vi "OAT Get Missing Pulses.vi"(3 "pulse positions":dbl[](array[numeric]) format="%.2f") -> (0 "pulses inserted":i32, 1 "modified pulse positions":dbl[](array[numeric]) format="%.2f")   [LabVIEW 2017, in "SoundVib_TachProcess.lvlib"]
uses:
  <vilib>/addons/Sound and Vibration/Order Analysis/Tach Process/SoundVib_TachProcess.lvlib
  <vilib>/Analysis/NI_AALBase.lvlib
panel:
  # "Get Missing Pules"
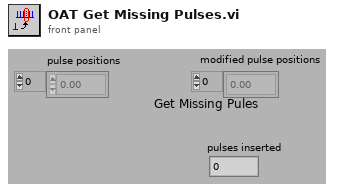
[diagram p1: front panel]
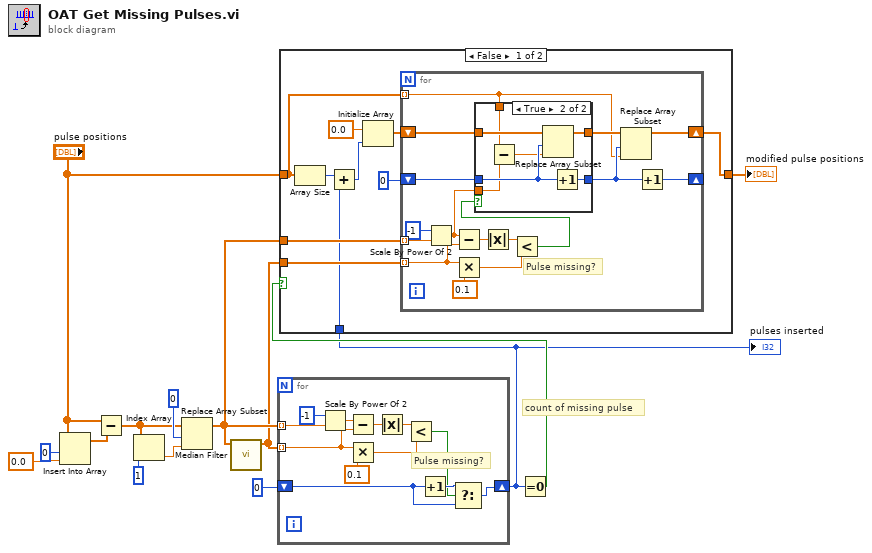
[diagram p0: block diagram]
diagram:
  # "count of missing pulse"
  n1 = Insert Into Array(array="pulse positions", index=0 ("Index"), new element=0.0) -> (w3:dbl[])
  n2 = Subtract(x="pulse positions", y=w3) -> (x-y=w1:dbl[])
  n3 = Index Array(array=w1, index=1 ("Index")) -> (element=w13:dbl)
  n4 = Replace Array Subset(array=w1, new element=w13, index=0 ("Index")) -> (w8:dbl[])
  n5 = call <vilib>:"Median Filter.vi"("X"=w8) -> ("Filtered X"=w7:dbl[])  [unwired: 9 in, 1 out]
  n6 = for {
    tunnel: w8 -> [w15] mode=indexing
    tunnel: w7 -> [w16] mode=indexing
    shift-right: [w26] -> w6
    shift-left: 0 -> [w24]
    # "Pulse missing?"
    n7 = Scale By Power Of 2(n=-1, x=w15) -> (x*2^n=w18:dbl)
    n8 = Subtract(x=w18, y=w16) -> (x-y=w23:dbl)
    n9 = Multiply(x=w16, y=0.1) -> (x*y=w20:dbl)
    n10 = Absolute Value(x=w23) -> (abs(x)=w22:dbl)
    n11 = Less?(x=w22, y=w20) -> (x < y?=w17:bool)
    n12 = Increment(x=w24) -> (x+1=w25:i32)
    n13 = Select(t=w25, s=w17, f=w24) -> (s? t:f=w26:i32)
  }
  "pulses inserted" <- w6
  n14 = Equal To 0?(x=w6) -> (x = 0?=w9:bool)
  n15 = case shown="False" w9 {
    tunnel: "pulse positions" -> [w28 w62]
    tunnel: [w29 w62] -> w10
    tunnel: w8 -> [w33 _]
    tunnel: w7 -> [w32 _]
    tunnel: w6 -> [w27 _]
    frame False {
      n16 = Array Size(array=w28) -> (size(s)=w35:i32)
      n17 = Add(x=w35, y=w27) -> (x+y=w34:i32)
      n18 = Initialize Array(0.0 ("Element Data"), w34) -> (w31:dbl[])
      n19 = for {
        tunnel: w33 -> [w45] mode=indexing
        tunnel: w32 -> [w44] mode=indexing
        shift-right: [w39] -> w29
        shift-left: w31 -> [w42]
        shift-right: [w41] -> _
        shift-left: 0 -> [w47]
        tunnel: w28 -> [w37] mode=indexing
        # "Pulse missing?"
        n20 = Scale By Power Of 2(n=-1, x=w45) -> (x*2^n=w43:dbl)
        n21 = Subtract(x=w43, y=w44) -> (x-y=w52:dbl)
        n22 = Multiply(x=w44, y=0.1) -> (x*y=w49:dbl)
        n23 = Absolute Value(x=w52) -> (abs(x)=w51:dbl)
        n24 = Less?(x=w51, y=w49) -> (x < y?=w48:bool)
        n25 = case shown="True" w48 {
          tunnel: [w54 w59] -> w40
          tunnel: w42 -> [w54 w60]
          tunnel: w47 -> [w53 w58]
          tunnel: [w53 w61] -> w38
          tunnel: w37 -> [_ w57]
          tunnel: w43 -> [_ w55]
          frame False {
          }
          frame True {
            n26 = Subtract(x=w57, y=w55) -> (x-y=w56:dbl)
            n27 = Replace Array Subset(array=w60, new element=w56, index=w58) -> (w59:dbl[])
            n28 = Increment(x=w58) -> (x+1=w61:i32)
          }
        }
        n29 = Replace Array Subset(array=w40, new element=w37, index=w38) -> (w39:dbl[])
        n30 = Increment(x=w38) -> (x+1=w41:i32)
      }
    }
    frame True {
    }
  }
  "modified pulse positions" <- w10
